vi "TagDB-Save.vi"(6 "version":string="my app 1.0", 8 "error in (no error)":errorcluster, 9 "ignore internal data(T)":bool=TRUE, 10 "file path(empty for default)":path, 11 "DB Ref":refnum<k1>) -> (0 "error out":errorcluster, 3 "DB Ref(dup)":refnum<k1>)   [LabVIEW 2017, in "TagDB.lvlib"]
doc: "[Covers: REQ_API_Save]"
uses:
  TagDB.lvlib
  _Support/Disk/tagdbfile-v3.1.ctl
  _Support/Error/_Build Error Cluster.vi
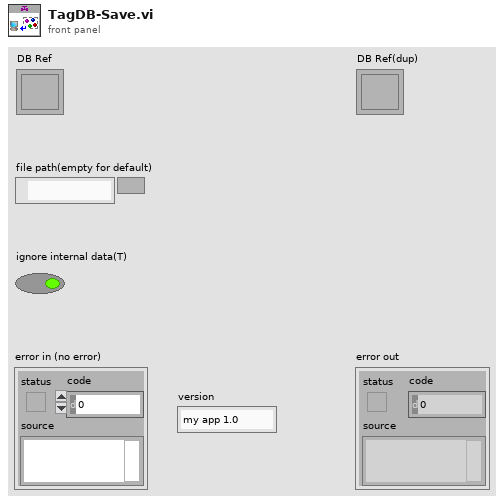
[diagram p1: front panel]
types:
  T1 = enum16{"open", "replace", "create", "open or create", "replace or create", "replace or create with confirmation"}
  T2 = typedef "TagDB.lvlib/tagdbfile-v3.1.ctl" = cluster{"version":string, "db":variant[]}
  T3 = typedef "TagDB.lvlib/tagdb-data.ctl" = cluster{"tag-map":variant, "timestamp-map":variant, "namecacher-map":variant, "DataTypeCacher-map":variant, "Tag Adding Lock?":bool, "Global Change Timestamp":timestamp, "Item Change Timestamp":timestamp, "name":string, "Global Change Flag":u64, "Item Change Flag":u64}
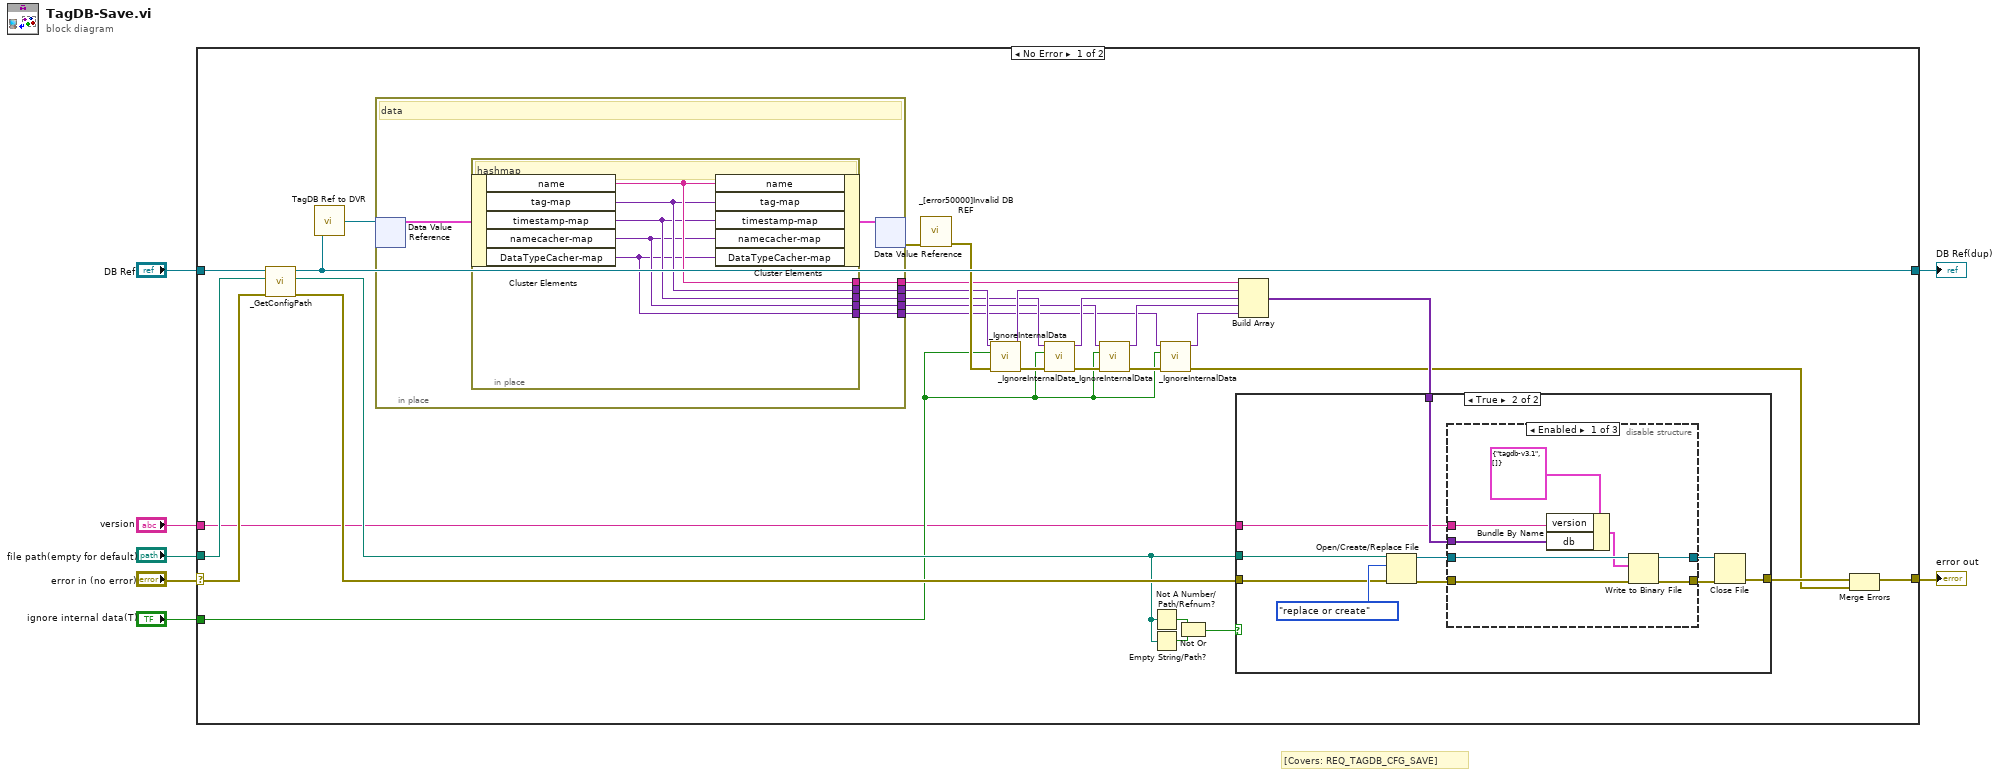
[diagram p0: block diagram]
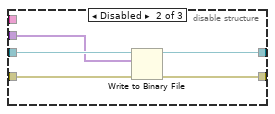
[diagram p3: hidden frame]
diagram:
  # "[Covers: REQ_TAGDB_CFG_SAVE]"
  n1 = case shown="No Error" "error in (no error)" {
    selector: "error in (no error)" -> [w33 w75]
    tunnel: [w28 w75] -> w6
    tunnel: [w34 w74] -> w4
    tunnel: "DB Ref" -> [w35 w74]
    tunnel: "file path(empty for default)" -> [w31 _]
    tunnel: "ignore internal data(T)" -> [w9 _]
    tunnel: "version" -> [w8 _]
    frame No Error {
      n2 = call "_GetConfigPath.vi"("error in (no error)"=w33, "file path(empty for default) in"=w31, "DB Ref"=w35) -> ("error out"=w32:errorcluster, "file path(empty for default) out"=w25:path, "DB Ref(dup)"=w34:refnum<k1>)  [unwired: 6 in]
      n3 = call "TagDB Ref to DVR.vi"("TagDB"=w34) -> ("DVR"=w36:refnum<data-value>)  [unwired: 4 in]
      n4 = in-place "In Place Element Structure" {
        in-place-border: [w66] -> w23
        in-place-border: [w65] -> w22
        in-place-border: [w64] -> w17
        in-place-border: [w63] -> w15
        in-place-border: [w62] -> w13
        # "data"
        n5 = in-place-dvr #1 ("Data Value Reference Read / Write Element")(w36) -> (w68:T3)  [unwired: 1 out]
        n6 = in-place "In Place Element Structure" {
          in-place-border: [w73] -> w66
          in-place-border: [w72] -> w65
          in-place-border: [w71] -> w64
          in-place-border: [w70] -> w63
          in-place-border: [w69] -> w62
          # "hashmap"
          n7 = in-place-cluster #2 ("Unbundle / Bundle Elements")(w68) -> ("name"=w73:string, "tag-map"=w72:variant, "timestamp-map"=w71:variant, "namecacher-map"=w70:variant, "DataTypeCacher-map"=w69:variant)
          n8 = in-place-cluster #2 ("Unbundle / Bundle Elements")("name"=w73, "tag-map"=w72, "timestamp-map"=w71, "namecacher-map"=w70, "DataTypeCacher-map"=w69) -> (w67:T3)
        }
        n9 = in-place-dvr #1 ("Data Value Reference Read / Write Element")(w67) -> (w30:errorcluster)  [unwired: 1 out]
      }
      n10 = call "_[error50000]Invalid DB REF.vi"("error in (no error)"=w30) -> ("error out"=w29:errorcluster)  [unwired: 10 in]
      n11 = call "_IgnoreInternalData.vi"("error in (no error)"=w29, "ignore internal data(T)"=w9, "Variant in"=w22) -> ("error out"=w21:errorcluster, "Variant out"=w18:variant)  [unwired: 7 in]
      n12 = call "_IgnoreInternalData.vi"("error in (no error)"=w21, "ignore internal data(T)"=w9, "Variant in"=w17) -> ("error out"=w20:errorcluster, "Variant out"=w16:variant)  [unwired: 7 in]
      n13 = call "_IgnoreInternalData.vi"("error in (no error)"=w20, "ignore internal data(T)"=w9, "Variant in"=w15) -> ("error out"=w19:errorcluster, "Variant out"=w14:variant)  [unwired: 7 in]
      n14 = Not A Number/Path/Refnum?(number/path/refnum=w25) -> (NaN/Path/Refnum?=w26:bool)
      n15 = Empty String/Path?(string/path=w25) -> (empty?=w27:bool)
      n16 = call "_IgnoreInternalData.vi"("error in (no error)"=w19, "ignore internal data(T)"=w9, "Variant in"=w13) -> ("error out"=w10:errorcluster, "Variant out"=w12:variant)  [unwired: 7 in]
      n17 = Not Or(1:w27, 2:w26) -> (0:w24:bool)
      n18 = Build Array(w23, w18, w16, w14, w12) -> (w11:variant[])
      n19 = case shown="True" w24 {
        tunnel: [w38 w48] -> w37
        tunnel: w11 -> [_ w40]
        tunnel: w32 -> [w38 w42]
        tunnel: w25 -> [_ w41]
        tunnel: w8 -> [_ w39]
        frame False {
        }
        frame True {
          n20 = Open/Create/Replace File(file path (use dialog)=w41, error in=w42, operation (0:open)=T1."replace or create") -> (refnum out=w45:refnum<file>, error out=w46:errorcluster)  [unwired: 3 in, 1 out]
          n21 = disable-structure shown="Enabled" {
            disable-tunnel: w46 -> [w56 w61 _]
            disable-tunnel: w45 -> [w55 w60 _]
            disable-tunnel: [w54 w59 _] -> w44
            disable-tunnel: [w53 w58 _] -> w43
            disable-tunnel: w40 -> [w51 w57 _]
            disable-tunnel: w39 -> [w49 _ _]
            frame Enabled {
              n22 = Bundle By Name(cluster=T2 {"version"="tagdb-v3.1", "db"=[]} ("tagdb-file-v3.1"), "version"=w49, "db"=w51) -> (w50:T2)
              n23 = Write to Binary File(file (use dialog)=w55, data=w50, error in=w56) -> (refnum out=w53:refnum<file>, error out=w54:errorcluster)  [unwired: 3 in, 1 out]
            }
            frame Disabled {
              n24 = Write to Binary File(file (use dialog)=w60, data=w57, error in=w61) -> (refnum out=w58:refnum<file>, error out=w59:errorcluster)  [unwired: 3 in, 1 out]
            }
            frame Disabled {
            }
          }
          n25 = Close File(refnum=w43, error in=w44) -> (error out=w48:errorcluster)  [unwired: 1 out]
        }
      }
      n26 = Merge Errors(w37, w10) -> (w28:errorcluster)
    }
    frame Error {
    }
  }
  "error out" <- w6
  "DB Ref(dup)" <- w4
